vi "Obtain Request Events.vi"(8 "error in (no error)":errorcluster, 10 "Create New? (F)":bool) -> (0 "error out":errorcluster, 2 "ZLG_CAN Request Events":T1)   [LabVIEW 2020, in "ZLG_CAN.lvlib"]
doc: "This VI Obtains/Creates the Requests events that will be used for other modules to communicate with the module that owns this VI. These Requests events will be accessed only via Public API methods for this module.\n\n<b>NOTE</b>: The contents of this VI are automatically generated and modified by the <b>Tools > Delacor > DQMH</b> utilities. Consider using those utilities instead of making your own modifications to this VI.\n_____\nBased on Delacor QMH Project Template 4.1.0.59."
uses:
  ZLG_CAN.lvlib
  Request Events--cluster.ctl
  Stop Argument--cluster.ctl
  Show Panel Argument--cluster.ctl
  Hide Panel Argument--cluster.ctl
  Get Module Execution Status Argument--cluster.ctl
  Show Diagram Argument--cluster.ctl
  Open_CAN Argument--cluster.ctl
  Init_CAN Argument--cluster.ctl
  Start_CAN Argument--cluster.ctl
  Start_CAN (Reply Payload)--cluster.ctl
  Sent_CAN Argument--cluster.ctl
  CAN_Frame.ctl
  Close_CAN Argument--cluster.ctl
  Reset_CAN Argument--cluster.ctl
  Recive_CAN Argument--cluster.ctl
  Recive_Wait Argument--cluster.ctl
  Recive_Wait (Reply Payload)--cluster.ctl
  CAN_OBJ_R.ctl
  Sent_Recive Argument--cluster.ctl
  Sent_Recive (Reply Payload)--cluster.ctl
panel:
  # "NOTE: The contents of this VI are automatically generated and modified by the Tools > Delacor > DQMH utilities. Consider using those utilities instead of making your own modifications to this VI."
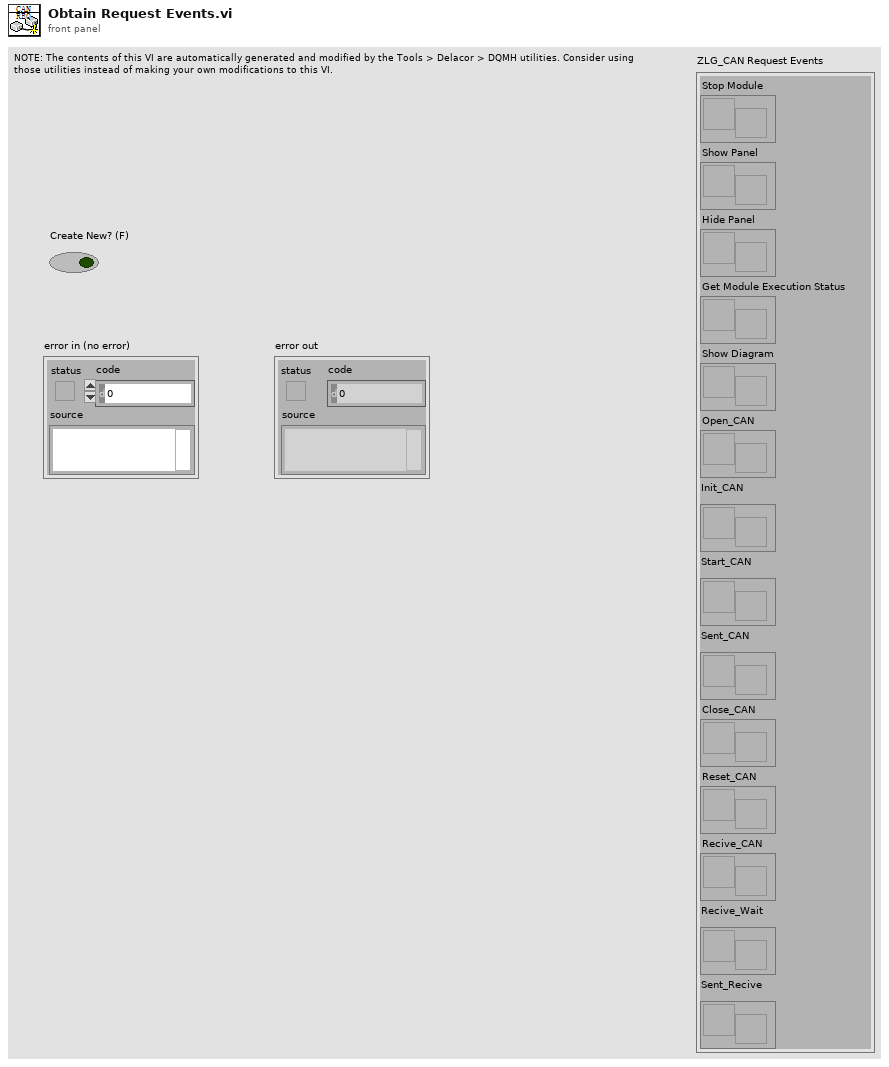
[diagram p1: front panel]
types:
  T1 = typedef "ZLG_CAN.lvlib/Request Events--cluster.ctl" = cluster{"Stop Module":refnum<user-event>, "Show Panel":refnum<user-event>, "Hide Panel":refnum<user-event>, "Get Module Execution Status":refnum<user-event>, "Show Diagram":refnum<user-event>, "Open_CAN":refnum<user-event>, "Init_CAN":refnum<user-event>, "Start_CAN":refnum<user-event>, "Sent_CAN":refnum<user-event>, "Close_CAN":refnum<user-event>, "Reset_CAN":refnum<user-event>, "Recive_CAN":refnum<user-event>, "Recive_Wait":refnum<user-event>, "Sent_Recive":refnum<user-event>}
  T2 = typedef "ZLG_CAN.lvlib/Sent_Recive Argument--cluster.ctl" = cluster{"ID":u32, "帧类型":u8, "帧格式":u8, "CAN_FRAME":T3, "帧长度":u8, "Wait Notifier":refnum<notifier>, "wait for reply":bool}
  T3 = typedef "ZLG_CAN.lvlib/CAN_Frame.ctl" = cluster{"[0]":u8, "[1]":u8, "[2]":u8, "[3]":u8, "[4]":u8, "[5]":u8, "[6]":u8, "[7]":u8}
  T4 = typedef "ZLG_CAN.lvlib/Recive_Wait Argument--cluster.ctl" = cluster{"Wait Notifier":refnum<notifier>, "wait for reply":bool}
  T5 = typedef "ZLG_CAN.lvlib/Recive_CAN Argument--cluster.ctl" = cluster{"布尔":bool}
  T6 = typedef "ZLG_CAN.lvlib/Reset_CAN Argument--cluster.ctl" = cluster{"设备类型":u32, "索引":u32, "CAN 通道":u32}
  T7 = typedef "ZLG_CAN.lvlib/Close_CAN Argument--cluster.ctl" = cluster{"设备类型":u32, "索引":u32}
  T8 = typedef "ZLG_CAN.lvlib/Sent_CAN Argument--cluster.ctl" = cluster{"ID":u32, "帧类型":u8, "帧格式":u8, "帧长度":u8, "CAN_FRAME":T3}
  T9 = typedef "ZLG_CAN.lvlib/Start_CAN Argument--cluster.ctl" = cluster{"布尔":bool, "Wait Notifier":refnum<notifier>, "wait for reply":bool}
  T10 = typedef "ZLG_CAN.lvlib/Init_CAN Argument--cluster.ctl" = cluster{"波特率":u32}
  T11 = typedef "ZLG_CAN.lvlib/Open_CAN Argument--cluster.ctl" = cluster{"设备类型":u32, "索引":u32, "CAN 通道":u32}
  T12 = typedef "ZLG_CAN.lvlib/Hide Panel Argument--cluster.ctl" = cluster{"Hide Panel?":bool}
  T13 = typedef "ZLG_CAN.lvlib/Show Panel Argument--cluster.ctl" = cluster{"Show Panel?":bool}
  T14 = typedef "ZLG_CAN.lvlib/Show Diagram Argument--cluster.ctl" = cluster{"Debug?":bool}
  T15 = typedef "ZLG_CAN.lvlib/Get Module Execution Status Argument--cluster.ctl" = cluster{"Running?":bool}
  T16 = typedef "ZLG_CAN.lvlib/Stop Argument--cluster.ctl" = cluster{"Origin":string, "Exit via Stop Module Req?":bool, "Wait for Module to stop?":bool}
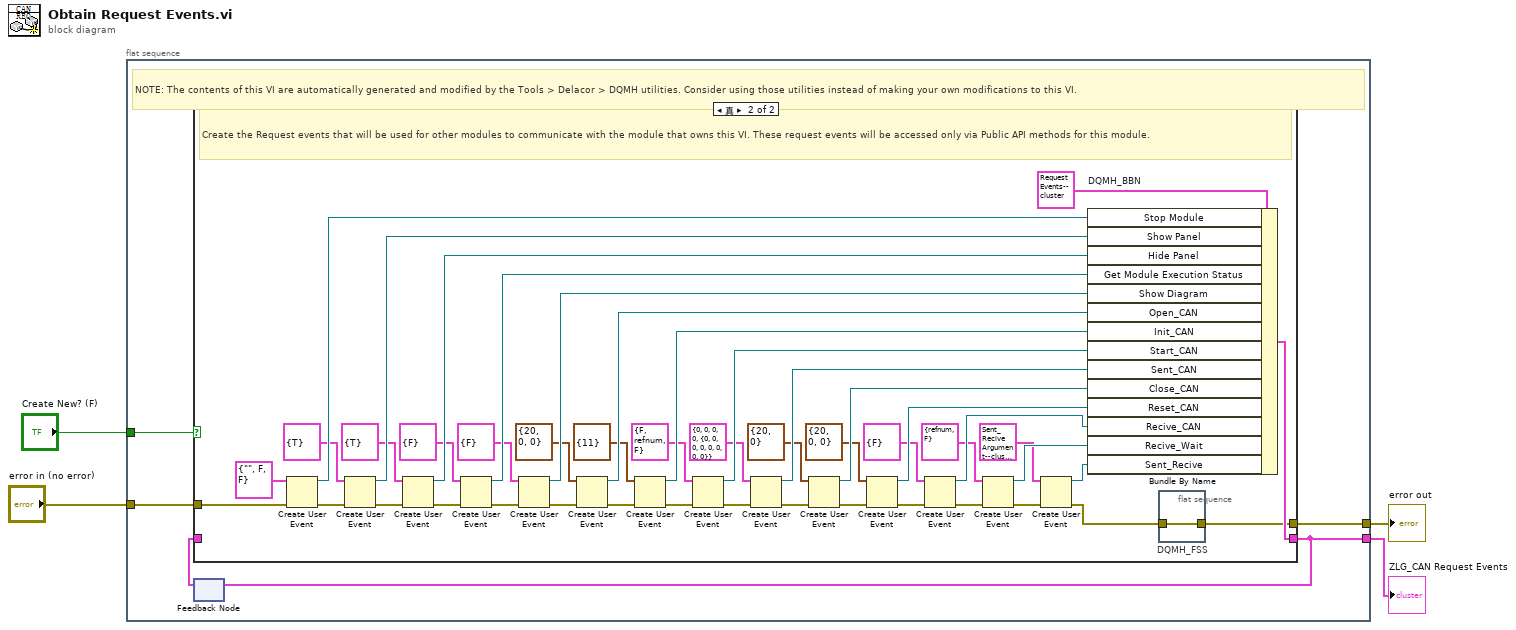
[diagram p0: block diagram]
diagram:
  n1 = flat-sequence {
    tunnel: [w9] -> w4
    tunnel: "error in (no error)" -> [w8]
    tunnel: [w6] -> w2
    tunnel: "Create New? (F)" -> [w5]
    frame #0 {
      # "NOTE: The contents of this VI are automatically generated and modified by the Tools > Delacor > DQMH utilities. Consider using those utilities instead of making your own modifications to this VI."
      n2 = feedback #1() -> (w7:T1)  [unwired: 1 in]
      n3 = case shown="真" w5 {
        tunnel: [w10 w47] -> w9
        tunnel: w8 -> [w10 w57]
        tunnel: [w11 w54] -> w6
        tunnel: w7 -> [w11 _]
        frame False {
          # "Obtain the Request events that were created in a previous call to this VI."
        }
        frame True {
          # "Create the Request events that will be used for other modules to communicate with the module that owns this VI. These request events will be accessed only via Public API methods for this module."
          n4 = Create User Event(user event datatype=T16 {"Origin"="", "Exit via Stop Module Req?"=FALSE, "Wait for Module to stop?"=FALSE} ("Stop Argument"), error in=w57) -> (user event=w55:refnum<user-event>, error out=w52:errorcluster)
          n5 = Create User Event(user event datatype=T13 {"Show Panel?"=TRUE} ("Show Panel Argument"), error in=w52) -> (user event=w51:refnum<user-event>, error out=w50:errorcluster)
          n6 = Create User Event(user event datatype=T12 {"Hide Panel?"=TRUE} ("Hide Panel Argument"), error in=w50) -> (user event=w49:refnum<user-event>, error out=w48:errorcluster)
          n7 = Create User Event(user event datatype=T15 {"Running?"=FALSE} ("Get Module Execution Status Argument"), error in=w48) -> (user event=w45:refnum<user-event>, error out=w46:errorcluster)
          n8 = Create User Event(user event datatype=T14 {"Debug?"=FALSE} ("Show Diagram Argument"), error in=w46) -> (user event=w42:refnum<user-event>, error out=w43:errorcluster)
          n9 = Create User Event(user event datatype=T11 {"设备类型"=20, "索引"=0, "CAN 通道"=0} ("Open_CAN Argument"), error in=w43) -> (user event=w37:refnum<user-event>, error out=w38:errorcluster)
          n10 = Create User Event(user event datatype=T10 {"波特率"=11} ("Init_CAN Argument"), error in=w38) -> (user event=w34:refnum<user-event>, error out=w35:errorcluster)
          n11 = Create User Event(user event datatype=T9 {"布尔"=FALSE, "Wait Notifier"=refnum, "wait for reply"=FALSE} ("Start_CAN Argument"), error in=w35) -> (user event=w31:refnum<user-event>, error out=w32:errorcluster)
          n12 = Create User Event(user event datatype=T8 {"ID"=0, "帧类型"=0, "帧格式"=0, "帧长度"=0, "CAN_FRAME"={"[0]"=0, "[1]"=0, "[2]"=0, "[3]"=0, "[4]"=0, "[5]"=0, "[6]"=0, "[7]"=0}} ("Sent_CAN Argument"), error in=w32) -> (user event=w28:refnum<user-event>, error out=w29:errorcluster)
          n13 = Create User Event(user event datatype=T7 {"设备类型"=20, "索引"=0} ("Close_CAN Argument"), error in=w29) -> (user event=w25:refnum<user-event>, error out=w26:errorcluster)
          n14 = Create User Event(user event datatype=T6 {"设备类型"=20, "索引"=0, "CAN 通道"=0} ("Reset_CAN Argument"), error in=w26) -> (user event=w22:refnum<user-event>, error out=w23:errorcluster)
          n15 = Create User Event(user event datatype=T5 {"布尔"=FALSE} ("Recive_CAN Argument"), error in=w23) -> (user event=w19:refnum<user-event>, error out=w20:errorcluster)
          n16 = Create User Event(user event datatype=T4 {"Wait Notifier"=refnum, "wait for reply"=FALSE} ("Recive_Wait Argument"), error in=w20) -> (user event=w16:refnum<user-event>, error out=w17:errorcluster)
          n17 = Create User Event(user event datatype=T2 {"ID"=0, "帧类型"=0, "帧格式"=0, "CAN_FRAME"={"[0]"=0, "[1]"=0, "[2]"=0, "[3]"=0, "[4]"=0, "[5]"=0, "[6]"=0, "[7]"=0}, "帧长度"=0, "Wait Notifier"=refnum, "wait for reply"=FALSE} ("Sent_Recive Argument"), error in=w17) -> (user event=w13:refnum<user-event>, error out=w14:errorcluster)
          n18 = Bundle By Name "DQMH_BBN"(cluster=T1 {"Stop Module"=refnum, "Show Panel"=refnum, "Hide Panel"=refnum, "Get Module Execution Status"=refnum, "Show Diagram"=refnum, "Open_CAN"=refnum, "Init_CAN"=refnum, "Start_CAN"=refnum, "Sent_CAN"=refnum, "Close_CAN"=refnum, "Reset_CAN"=refnum, "Recive_CAN"=refnum, "Recive_Wait"=refnum, "Sent_Recive"=refnum} ("output cluster"), "Stop Module"=w55, "Show Panel"=w51, "Hide Panel"=w49, "Get Module Execution Status"=w45, "Show Diagram"=w42, "Open_CAN"=w37, "Init_CAN"=w34, "Start_CAN"=w31, "Sent_CAN"=w28, "Close_CAN"=w25, "Reset_CAN"=w22, "Recive_CAN"=w19, "Recive_Wait"=w16, "Sent_Recive"=w13) -> (w54:T1)
          n19 = flat-sequence "DQMH_FSS" {
            tunnel: w14 -> [w58]
            tunnel: [w58] -> w47
            frame #0 {
            }
          }
        }
      }
      n20 = feedback-in #1(w6) -> ()
    }
  }
  "ZLG_CAN Request Events" <- w2
  "error out" <- w4
